vi "VisRequestOverride.vi"(8 "Error in":errorcluster[](array[cluster]), 11 "Visualize":refnum<class "VisualizeBase.lvclass">) -> (0 "Error out":errorcluster[](array[cluster]), 3 "RequestEvents":T1)   [LabVIEW 2018, in "Visualization.lvlib" / "VisualizeBase.lvclass"]
uses:
  VisualizeBase.lvclass
  VisRequestEvents.ctl
  VisUserEventType.ctl
  <userlib>/NIST/NISTErrorLib/NISTErrorLib.lvlib
panel:
  # "This dynamic terminal makes the vi overridable and is marked in the base class as \"Must Override\".  \n\nSo any child class derived from this parent class must override this VI"
  # "If you want to add other Request Events, open this typedef, copy an existing event and rename it to your event name."
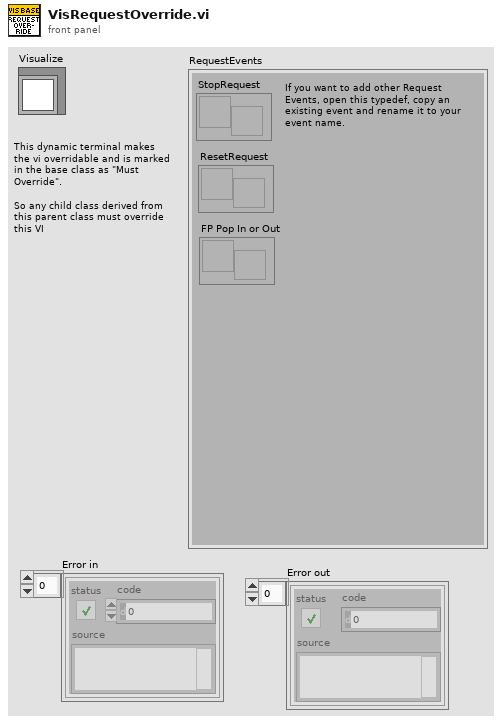
[diagram p1: front panel]
types:
  T1 = typedef "Visualization.lvlib/VisualizeBase.lvclass/VisRequestEvents.ctl" = cluster{"StopRequest":refnum<user-event>, "ResetRequest":refnum<user-event>, "FP Pop In or Out":refnum<user-event>}
  T2 = typedef "Visualization.lvlib/VisualizeBase.lvclass/clRequestEvents.ctl" = cluster{"StopRequest":refnum<user-event>, "ResetRequest":refnum<user-event>, "FP Pop In or Out":refnum<user-event>}
  T3 = typedef "Visualization.lvlib/VisualizeBase.lvclass/VisUserEventType.ctl" = cluster{"BusIndex":i8, "Data":variant}
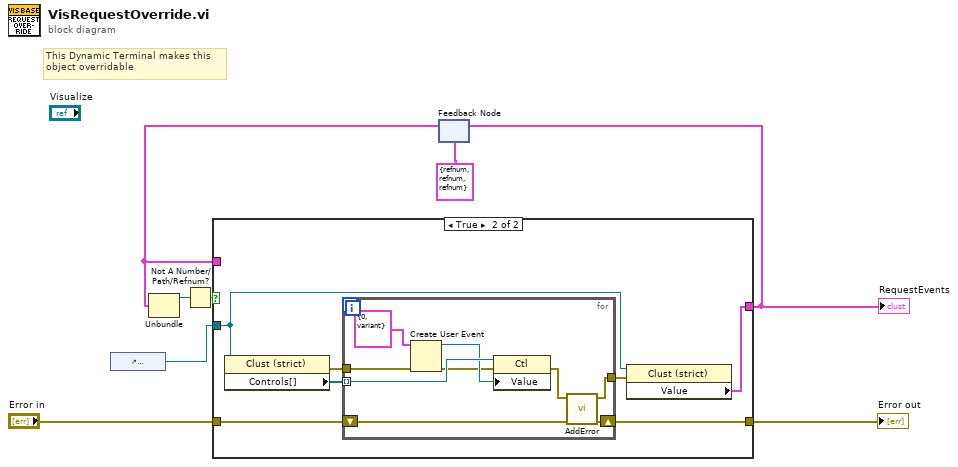
[diagram p0: block diagram]
diagram:
  # "This Dynamic Terminal makes this\nobject overridable"
  n1 = control-ref of="RequestEvents"() -> (w1:refnum<vi>)
  n2 = feedback #1(T1 {"StopRequest"=refnum, "ResetRequest"=refnum, "FP Pop In or Out"=refnum} ("Value")) -> (w6:T2)
  n3 = Unbundle(w6) -> ("StopRequest"=w8:refnum<user-event>)  [unwired: 2 out]
  n4 = Not A Number/Path/Refnum?(number/path/refnum=w8) -> (NaN/Path/Refnum?=w7:bool)
  n5 = case shown="True" w7 {
    tunnel: [w10 w12] -> w2
    tunnel: w6 -> [w10 _]
    tunnel: [w9 w14] -> w4
    tunnel: "Error in" -> [w9 w15]
    tunnel: w1 -> [_ w11]
    frame False {
    }
    frame True {
      n6 = property on="Property Node" class="Clust (strict)"(reference=w11) -> (error out=w16:errorcluster, "Controls[]"=w17:refnum<vi>[])  [unwired: 1 in, 1 out]
      n7 = for {
        tunnel: w17 -> [w24] mode=indexing
        tunnel: w16 -> [w25]
        shift-right: [w19] -> w14
        shift-left: w15 -> [w20]
        tunnel: [w18] -> w13
        n8 = Create User Event(user event datatype=T3 {"BusIndex"=0, "Data"=variant} ("clEventType"), error in=w25) -> (user event=w23:refnum<user-event>, error out=w22:errorcluster)
        n9 = property class="Ctl"(reference=w24, error in=w22, "Value"=w23) -> (error out=w21:errorcluster)  [unwired: 1 out]
        n10 = call <userlib>:"AddError.vi"("ErrorArray In"=w20, "error in (no error)"=w21) -> ("ErrorArray Out"=w19:errorcluster[], "error out"=w18:errorcluster)  [unwired: 8 in]
      }
      n11 = property on="Property Node" class="Clust (strict)"(reference=w11, error in=w13) -> ("Value"=w12:T2)  [unwired: 2 out]
    }
  }
  "Error out" <- w4
  "RequestEvents" <- w2
  n12 = feedback-in #1(w2) -> ()
